vi "Stage_2_waveform_for_DAQ.vi"(11 "input cluster":T2) -> (2 "DAQ cluster":T1, 3 "time cluster":cluster{"total time":dbl, "time per step":dbl})   [LabVIEW 2016]
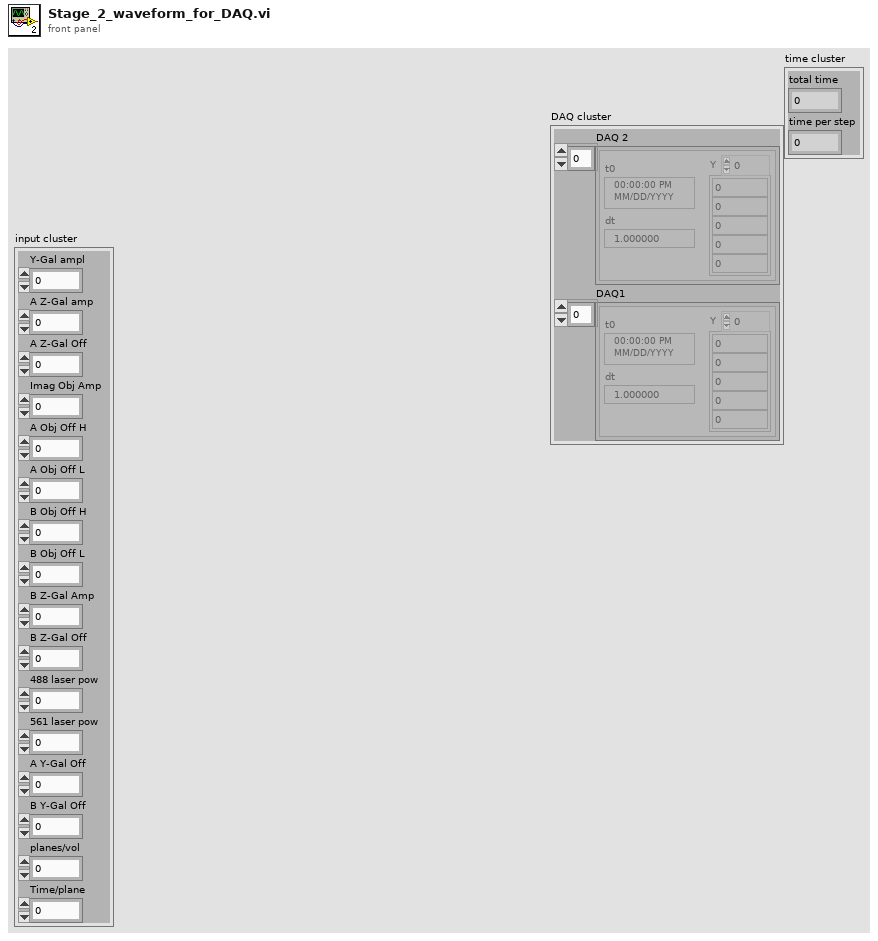
[diagram p1: front panel]
types:
  T1 = cluster{"DAQ1":waveform(dbl)[], "DAQ 2":waveform(dbl)[]}
  T2 = cluster{"Y-Gal ampl":dbl, "A Z-Gal amp":dbl, "A Z-Gal Off":dbl, "Imag Obj Amp":dbl, "A Obj Off H":dbl, "A Obj Off L":dbl, "B Obj Off H":dbl, "B Obj Off L":dbl, "B Z-Gal Amp":dbl, "B Z-Gal Off":dbl, "488 laser pow":dbl, "561 laser pow":dbl, "A Y-Gal Off":dbl, "B Y-Gal Off ":dbl, "planes/vol":dbl, "Time/plane":dbl}
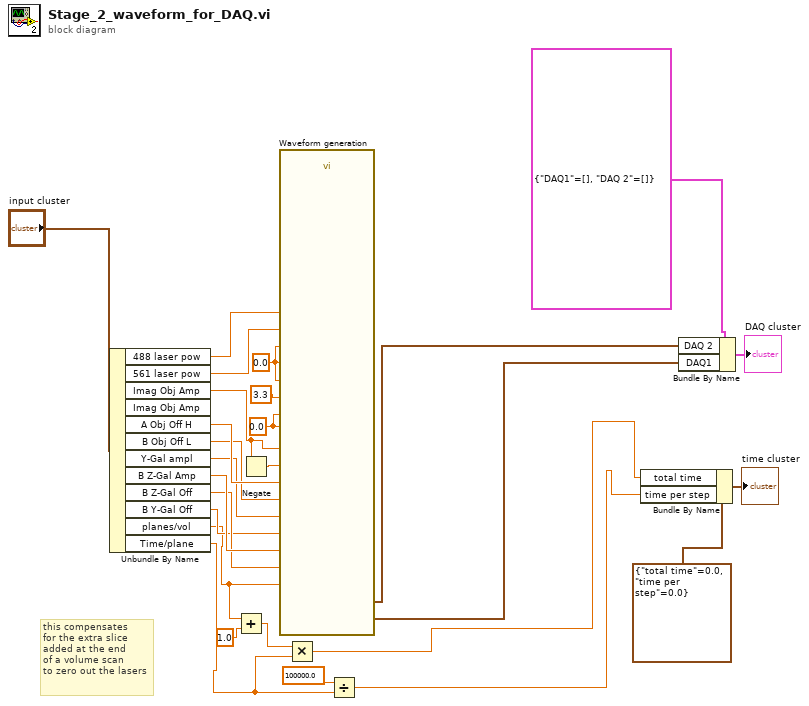
[diagram p0: block diagram]
diagram:
  w24 = 0.0 ("SPIMB Camera Trigger")
  w25 = 0.0 ("ARM1 Y-Galvo Offset")
  # "this compensates\nfor the extra slice\nadded at the end\nof a volume scan\nto zero out the lasers"
  n1 = Unbundle By Name("input cluster") -> ("488 laser pow"=w16:dbl, "561 laser pow"=w17:dbl, "Imag Obj Amp"=w14:dbl, "A Obj Off H"=w23:dbl, "B Obj Off L"=w22:dbl, "Y-Gal ampl"=w20:dbl, "B Z-Gal Amp"=w21:dbl, "B Z-Gal Off"=w19:dbl, "B Y-Gal Off"=w15:dbl, "planes/vol"=w11:dbl, "Time/plane"=w13:dbl)  [unwired: 1 out]
  n2 = Add(x=w11, y=1.0) -> (x+y=w12:dbl)
  n3 = Negate(x=w14) -> (-x=w18:dbl)
  n4 = call "Waveform generation.vi"("Number of Steps"=w11, "488 LASER Intensity"=w16, "SPIMA Obj Ampl"=w14, "SPIMB Z- galvo amplitude"=w21, "SPIMA Z-Galvo Offset"=w25, "SPIMA Z-Galvo Amplitude"=w25, "SPIMA Camera trigger"=3.3 ("ARM2 Camera trigger"), "SPIMA Objective Offset"=w23, "SPIMB Objective Offset"=w22, "SPIMA Y-Galvo Offset"=w24, "SPIMB Camera Trigger"=w24, "561 Laser Amplitude"=w17, "SPIMB Objective Amplitude"=w18, "SPIMA Y-Galvo Amplitude"=w24, "SPIMB Z-offset"=w19, "SPIMB Y Offset"=w15, "SPIMB Y Amplitude"=w20) -> ("DAQ 2"=w7:waveform(dbl)[], "DAQ1"=w6:waveform(dbl)[])  [unwired: 9 in]
  n5 = Multiply(x=w12, y=w13) -> (x*y=w3:dbl)
  n6 = Divide(x=100000.0, y=w13) -> (x/y=w2:dbl)
  n7 = Bundle By Name(cluster=cluster{"total time":dbl, "time per step":dbl} {"total time"=0.0, "time per step"=0.0}, "total time"=w3, "time per step"=w2) -> (→"time cluster":cluster{"total time":dbl, "time per step":dbl})
  n8 = Bundle By Name(cluster=T1 {"DAQ1"=[], "DAQ 2"=[]}, "DAQ 2"=w7, "DAQ1"=w6) -> (→"DAQ cluster":T1)
